vi "Is Read Only.vi"(8 "Error In":errorcluster, 11 "Dual Mode Thermometer in":refnum<class "Dual Mode Thermometer.lvclass">) -> (0 "Error Out":errorcluster, 2 "Read Only":bool, 3 "Dual Mode Thermometer out":refnum<class "Dual Mode Thermometer.lvclass">)   [LabVIEW 2014, in "Dual Mode Thermometer.lvclass"]
doc: "Checks if this thermometer is user-editable (False) or read-only (True).\n\n\nCopyright (c) 2019 Sze Howe Koh.\nThis code is licensed under the MIT license."
uses:
  Dual Mode Thermometer.lvclass
  Dual Mode Thermometer.lvclass/Dual Mode Thermometer.ctl
  <vilib>/addons/LQ/Qt Widgets/QWidget/QWidget.lvclass
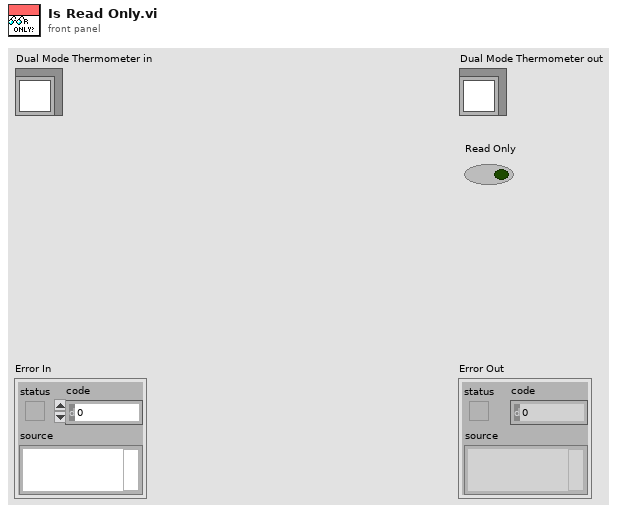
[diagram p1: front panel]
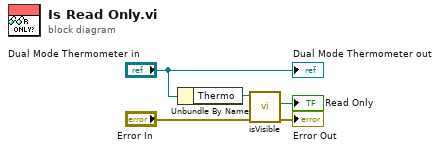
[diagram p0: block diagram]
diagram:
  n1 = Unbundle By Name("Dual Mode Thermometer in") -> ("Thermo"=w4:refnum<class "QwtThermo.lvclass">)
  n2 = call <vilib>:"isVisible.vi"("Error In"="Error In", "QWidget In"=w4) -> ("Error Out"=→"Error Out":errorcluster, "Value"=→"Read Only":bool)  [unwired: 7 in, 1 out]
  "Dual Mode Thermometer out" <- "Dual Mode Thermometer in"
